vi "TMC_Queue_Commands.vi"(1 "TMC-Control":T1, 3 "TMC Queue":refnum<queue>) -> (0 "TMC-Control new":T1)   [LabVIEW 2019]
uses:
  Torque_TMC/TMC_Control.ctl
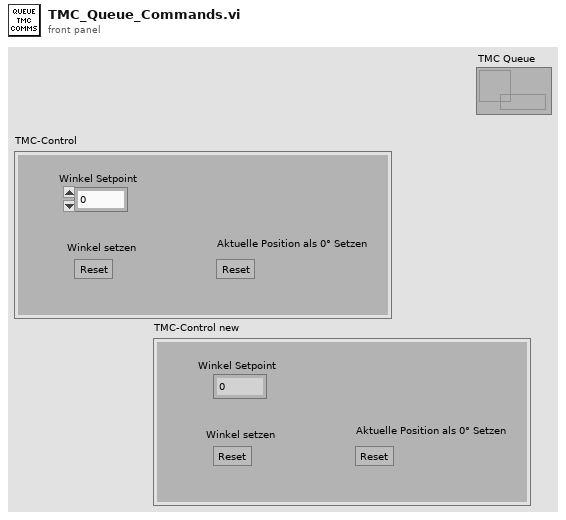
[diagram p1: front panel]
types:
  T1 = typedef "TMC_Control.ctl" = cluster{"Winkel Setpoint":dbl, "Aktuelle Position als 0° Setzen":bool, "Winkel setzen":bool}
  T2 = cluster{"Winkel Setpoint":bool, "Aktuelle Position als 0° Setzen":bool, "Winkel setzen":bool}
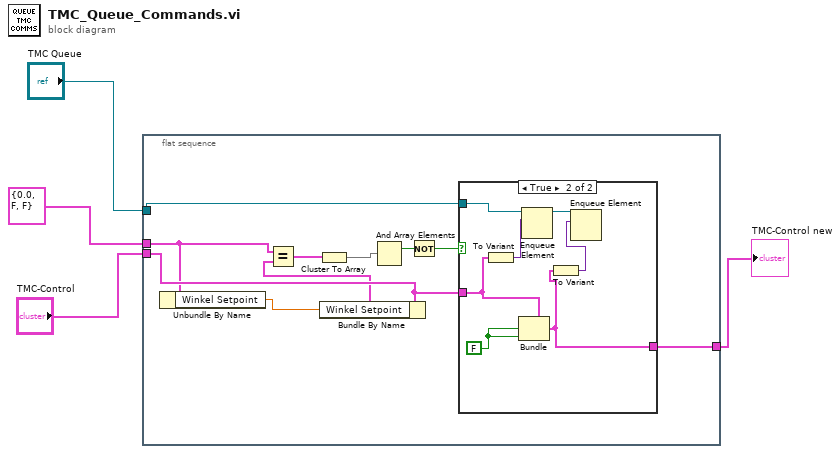
[diagram p0: block diagram]
diagram:
  n1 = flat-sequence {
    tunnel: "TMC Queue" -> [w14]
    tunnel: "TMC-Control" -> [w9]
    tunnel: T1 {"Winkel Setpoint"=0.0, "Aktuelle Position als 0° Setzen"=FALSE, "Winkel setzen"=FALSE} ("TMC-Control 2") -> [w7]
    tunnel: [w10] -> w1
    frame #0 {
      n2 = Unbundle By Name(w7) -> ("Winkel Setpoint"=w6:dbl)
      n3 = Bundle By Name(cluster=w9, "Winkel Setpoint"=w6) -> (w8:T1)
      n4 = Equal?(x=w7, y=w8) -> (x = y?=w5:T2)
      n5 = Cluster To Array(cluster=w5) -> (array=w13:bool[])
      n6 = And Array Elements(Boolean array=w13) -> (logical AND=w12:bool)
      n7 = Not(x=w12) -> (.not. x?=w11:bool)
      n8 = case shown="True" w11 {
        tunnel: w14 -> [_ w22]
        tunnel: w9 -> [w15 w18]
        tunnel: [w15 w17] -> w10
        frame False {
        }
        frame True {
          w16 = FALSE
          n9 = To Variant(anything=w18) -> (Variant=w21:variant)
          n10 = Bundle(cluster=w18, "Aktuelle Position als 0° Setzen"=w16, "Winkel setzen"=w16) -> (w17:T1)  [unwired: 1 in]
          n11 = Enqueue Element(queue=w22, element=w21) -> (queue out=w20:refnum<queue>)  [unwired: 2 in, 2 out]
          n12 = To Variant(anything=w17) -> (Variant=w19:variant)
          n13 = Enqueue Element(queue=w20, element=w19) -> ()  [unwired: 2 in, 3 out]
        }
      }
    }
  }
  "TMC-Control new" <- w1
